vi "Keithley 6517A Scanner Control.vi"(1 "Scan List":string="1,2,3,4,5,6,7,8,9,10", 2 "Open / Close Internal Scanner Channel":i16=1 min=1 max=10 step=1, 3 "error in":T1, 4 "Scanner Control":u16(ring) items=["Open All", "Open Channel", "Close Channel", "Scan List"], 5 "GPIB address":string="27") -> (0 "error out":T1)   [LabVIEW 2024]
doc: "This VI is used to set up the 6517A for internal scanning only using the 6521 or 6522 scanner boards.\n\nScanner Control\n0 = Open All\n1 = Open Channel\n2 = Close Channel\n3 = Scan List\n\nThe scan list must have the channels in continguous order. For example to scan channels 1 through 10, the scan list would be:\n1,2,3,4,5,6,7,8,9,10\nIf the you want to scan channels 1, 4, 7, 9, 10, the scan list would be: 1,4,7,9,10"
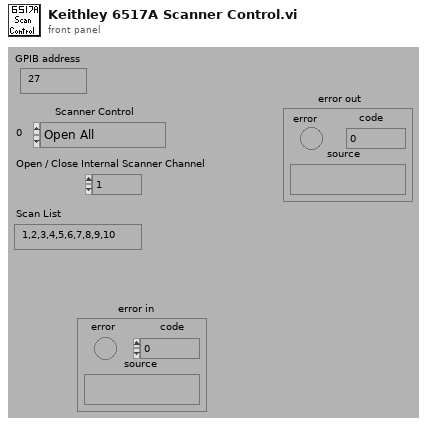
[diagram p1: front panel]
types:
  T1 = cluster{"error":bool, "code":i32, "source":string}
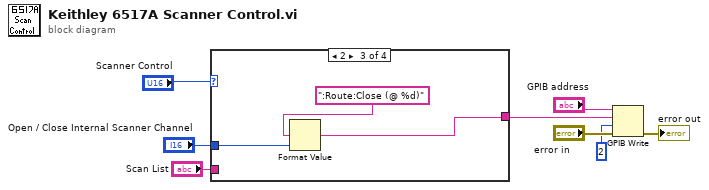
[diagram p0: block diagram]
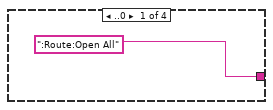
[diagram p2: hidden frame]
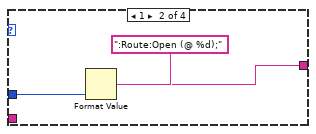
[diagram p3: hidden frame]
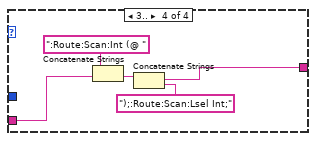
[diagram p4: hidden frame]
diagram:
  n1 = case shown="2" "Scanner Control" {
    tunnel: [":Route:Open All" w10 w13 w16] -> w4
    tunnel: "Open / Close Internal Scanner Channel" -> [_ w11 w14 _]
    tunnel: "Scan List" -> [_ _ _ w19]
    frame ..0 {
    }
    frame 1 {
      n2 = Format Value(format string=":Route:Open (@ %d);", value (0)=w11) -> (output string=w10:string)  [unwired: 1 in]
    }
    frame 2 {
      n3 = Format Value(format string=":Route:Close (@ %d)", value (0)=w14) -> (output string=w13:string)  [unwired: 1 in]
    }
    frame 3.. {
      n4 = Concatenate Strings(":Route:Scan:Int (@ ", w19) -> (w18:string)
      n5 = Concatenate Strings(w18, ");:Route:Scan:Lsel Int;") -> (w16:string)
    }
  }
  n6 = GPIB Write(0:"GPIB address", 1:w4, 2:2, 3:"error in") -> (6:→"error out":errorcluster)  [unwired: 1 in, 1 out]
